vi "FITS_HDR-extr-param.VI"(0 "Parameter sel":u16(ring) items=["SIMPLE", "BITPIX", "NAXIS", "NAXIS1", "NAXIS2", "extend", "fowlernumber", "object", "telescope", "instrument", "observer", "equinox", "name", "date", "time", "Julian", "inttime", "filter", "bscale", "bzero", "ctype1", "ctype2", "crval1", "crval2", "crpix1", "crpix2", "tempA", "tempB", "tempc1", "tempc2", "tempc3", "tempc4", "tempd1", "tempd2", "tempd3", "tempd4", "bias1", "bias2", "bias3", "bias4", "bias5", "bias6", "bias7", "bias8", "focus1", "focus2", "focus3", "fltindx", "fltstep", "fname", "pressure", "heat1", "heat2", "heatd"], 1 "Header in":string, 2 "PARAM type?":u16(ring) items=["Numeric", "Text string"], 3 "Error In":errorcluster, 4 "Param value to write":string, 5 "Param name":string="c:\\DATA") -> (7 "HDR PARAM txt string":string, 9 "HDR PARAM Value":dbl, 10 "Error Out":errorcluster)   [LabVIEW 2017]
uses:
  <userlib>/_FITS_RW/FITS Header Global.vi
panel:
  in  "Write?":bool
  out "HDR PARAM Value 2":dbl
  out "Hdr param value (string)":string
  out "String Array Selected":string[](array[string])=["c:\\DATA\\20141011-102717-0.fits", "c:\\DATA\\20141011-102717-1.fits"]
  out "HEADER LABELS":string[](array[string])=["SIMPLE", "BITPIX", "NAXIS", "NAXIS1", "NAXIS2", "extend", "fowlernumber", "object", "telescope", "instrument", "observer", "equinox", "name", "date", "time", "Julian", "inttime", "filter", "bscale", "bzero", "ctype1", "ctype2", "crval1", "crval2", "crpix1", "crpix2", "tempA", "tempB", "tempc1", "tempc2", "tempc3", "tempc4", "tempd1", "tempd2", "tempd3", "tempd4", "bias1", "bias2", "bias3", "bias4", "bias5", "bias6", "bias7", "bias8", "focus1", "focus2", "focus3", "fltindx", "fltstep", "fname", "pressure", "heat1", "heat2", "heatd"]
  in  "HDR PARAM name":string
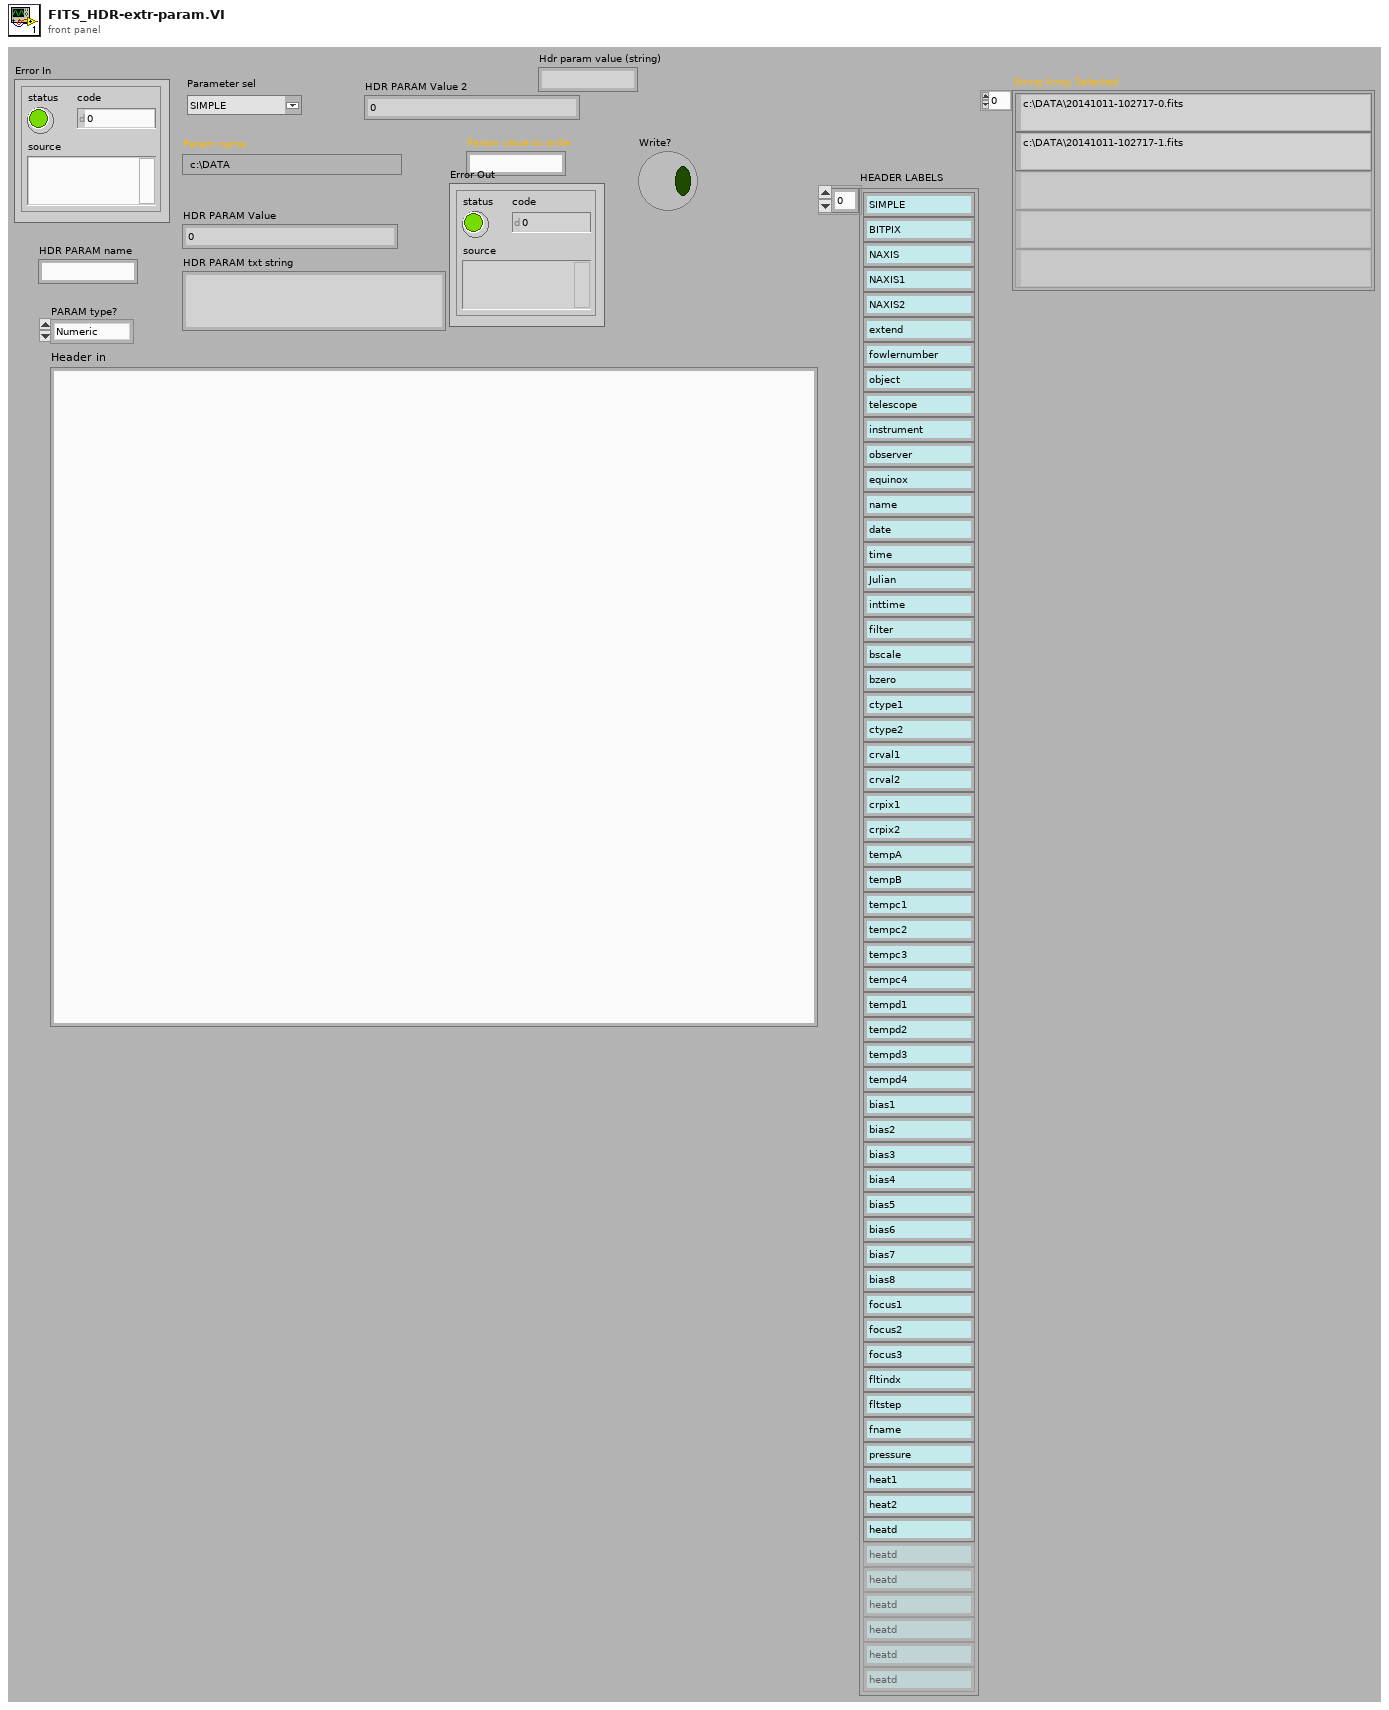
[diagram p1: front panel]
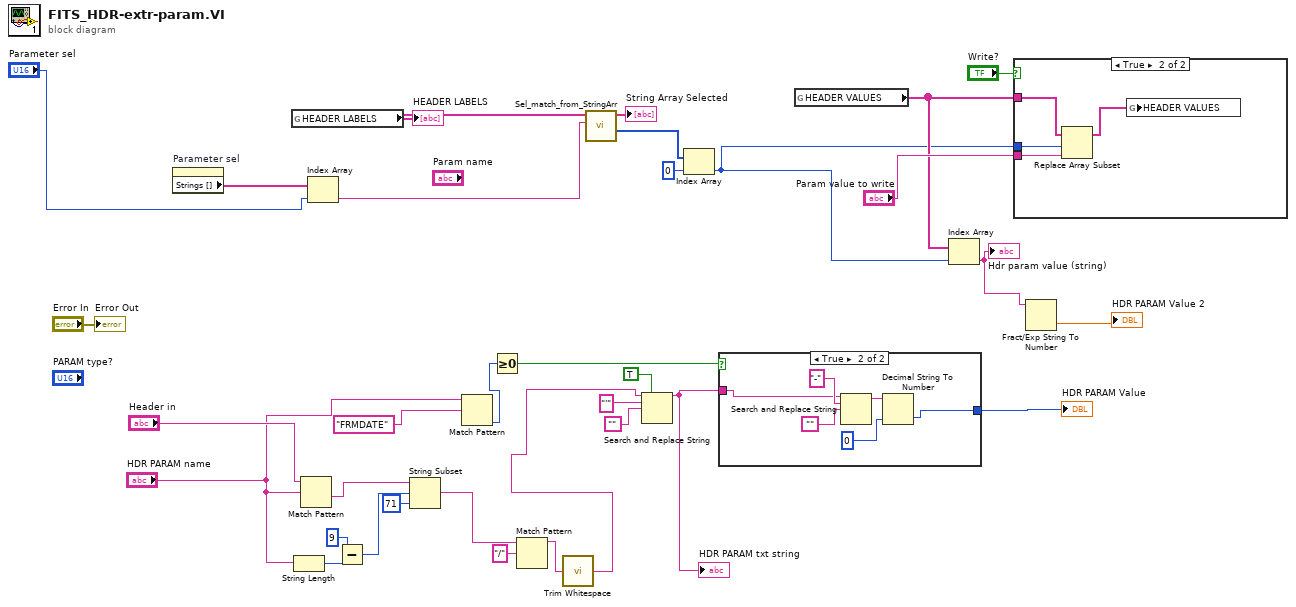
[diagram p0: block diagram]
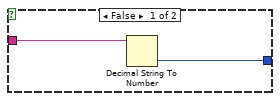
[diagram p3: hidden frame]
diagram:
  n1 = property on="Parameter sel" class="Ring (strict)"() -> ("Strings []"=w10:string[])  [unwired: 2 in, 2 out]
  n2 = global read "FITS Header Global.vi" "HEADER LABELS"() -> (w11:string[])
  "HEADER LABELS" <- w11
  n3 = String Length(string="HDR PARAM name") -> (length=w30:i32)
  n4 = Match Pattern(string="Header in", regular expression="HDR PARAM name") -> (after substring=w29:string)  [unwired: 1 in, 3 out]
  n5 = Index Array(array=w10, index="Parameter sel") -> (element=w8:string)
  n6 = Subtract(x=9, y=w30) -> (x-y=w32:i32)
  n7 = String Subset(string=w29, offset (0)=w32, length (rest)=71 ("length (rest)")) -> (substring=w23:string)
  n8 = Match Pattern(string="HDR PARAM name", regular expression="FRMDATE") -> (offset past match=w21:i32)  [unwired: 1 in, 3 out]
  n9 = Greater Or Equal To 0?(x=w21) -> (x >= 0?=w20:bool)
  n10 = Match Pattern(string=w23, regular expression="/") -> (before substring=w27:string)  [unwired: 1 in, 3 out]
  n11 = call <vilib>:"Trim Whitespace.vi"("string"=w27) -> ("trimmed string"=w16:string)  [unwired: 1 in]
  n12 = call <userlib>:"Sel_match_from_StringArr.vi"("String to match"=w8, "String Array In"=w11) -> ("Inx Exact match"=w1:i32[], "String Array Matched"=→"String Array Selected":string[])  [unwired: 5 in, 3 out]
  n13 = Search and Replace String(replace all?=TRUE ("replace all? (F)"), input string=w16, search string="'", replace string="") -> (result string=w15:string)  [unwired: 4 in, 3 out]
  "HDR PARAM txt string" <- w15
  n14 = Index Array(array=w1, index=0) -> (element=w5:i32)
  n15 = case shown="True" w20 {
    tunnel: [w35 w39] -> w24
    tunnel: w15 -> [w34 w36]
    frame False {
      n16 = Decimal String To Number(string=w34) -> (number=w35:i32)  [unwired: 2 in, 1 out]
    }
    frame True {
      n17 = Search and Replace String(input string=w36, search string="-", replace string="") -> (result string=w40:string)  [unwired: 5 in, 3 out]
      n18 = Decimal String To Number(string=w40, default (0L)=i64 0) -> (number=w39:i64)  [unwired: 1 in, 1 out]
    }
  }
  "HDR PARAM Value" <- w24
  n19 = global read "FITS Header Global.vi" "HEADER VALUES"() -> (w6:string[])
  n20 = Index Array(array=w6, index=w5) -> (element=w4:string)
  "Hdr param value (string)" <- w4
  n21 = case shown="True" "Write?" {
    tunnel: "Param value to write" -> [_ w44]
    tunnel: w6 -> [_ w43]
    tunnel: w5 -> [_ w42]
    frame False {
    }
    frame True {
      n22 = Replace Array Subset(array=w43, new element=w44, index=w42) -> (w45:string[])
      n23 = global write "FITS Header Global.vi" "HEADER VALUES"(w45) -> ()
    }
  }
  n24 = Fract/Exp String To Number(string=w4) -> (number=→"HDR PARAM Value 2":dbl)  [unwired: 3 in, 1 out]
  "Error Out" <- "Error In"
